vi "TeachableMachines.vi"() -> ()   [LabVIEW 2020]
uses:
  EN1Course-master/_Subs/SystemLink/SL_Subs/SL_XControl.xctl
  EN1Course-master/_Subs/SystemLink/SL_Subs/SystemLink_Write_String.vi
panel:
  in  "Image Path":path
  in  "Path to keras folder":path
  in  "Ask":bool
  in  "stop":bool
  out "dt":u32=141
  out "picture":picture
  out "Percentages":u8[](array[slide])=[0, 99, 1, 0] scale=0.0..100.0
  out "Labels":string="0 go\n1 stop\n2 right\n3 nothing\n"
  in  "SystemLink":T1(xcontrol)
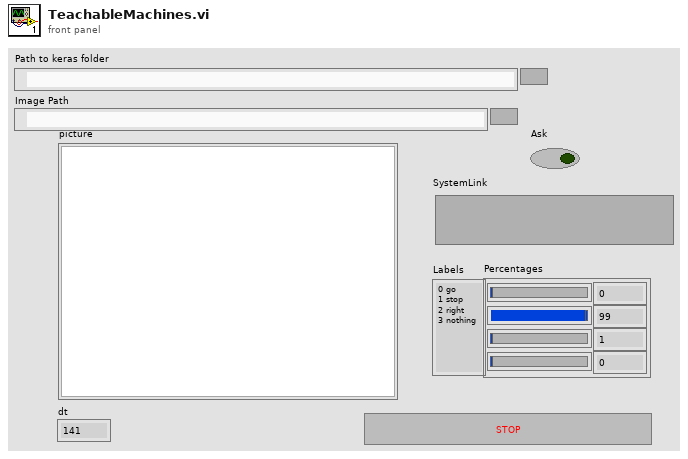
[diagram p1: front panel]
types:
  T1 = cluster{"Tag":string, "Type":string, "Data":string}
  T2 = cluster{"session":refnum<k35>, "Tensor Flow":path, "Image":path, "Labels":string}
  T3 = typedef "imagedata.ctl" = cluster{"image type":i32, "image depth":i32, "image":u8[], "mask":u8[], "colors":u32[], "Rectangle":cluster{"left":i16, "top":i16, "right":i16, "bottom":i16}}
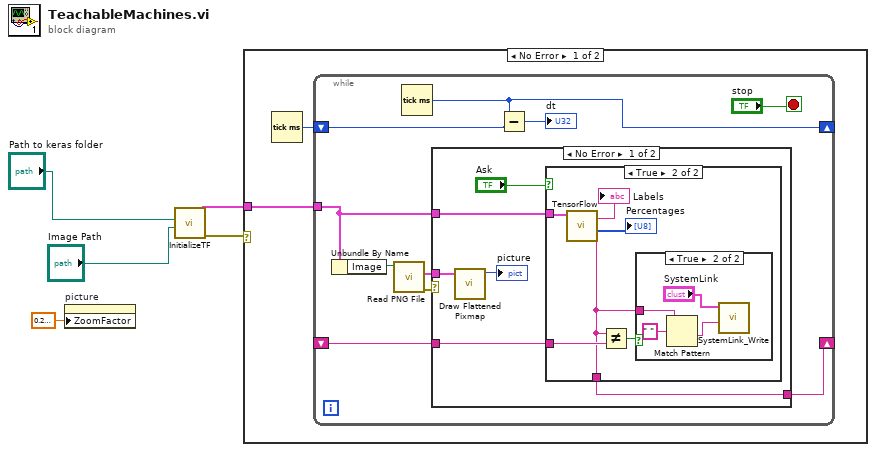
[diagram p0: block diagram]
diagram:
  n1 = property on="picture" class="Pict"("ZoomFactor"=sgl 0.2 ("Zoom Factor")) -> ()  [unwired: 2 in, 2 out]
  n2 = call "InitializeTF.vi"("Image Path"="Image Path", "Path to keras folder"="Path to keras folder") -> ("error out"=w4:errorcluster, "TFinfo out"=w5:T2)  [unwired: 8 in]
  n3 = case shown="No Error" w4 {
    tunnel: w5 -> [w7 _]
    frame No Error {
      n4 = Tick Count (ms)() -> (millisecond timer value=w6:u32)
      n5 = while {
        tunnel: w7 -> [w11]
        shift-right: [w17] -> _
        shift-left: w6 -> [w16]
        shift-right: [w12] -> _
        shift-left: _ -> [w13]
        stop <- "stop" stop-if-true
        n6 = Unbundle By Name(w11) -> ("Image"=w10:path)
        n7 = call <vilib>:"Read PNG File.vi"("path to PNG file"=w10) -> ("error out"=w8:errorcluster, "image data"=w9:T3)  [unwired: 8 in, 1 out]
        n8 = Tick Count (ms)() -> (millisecond timer value=w17:u32)
        n9 = case shown="No Error" w8 {
          tunnel: w13 -> [w23 w35]
          tunnel: [w22 w35] -> w12
          tunnel: w11 -> [w21 _]
          tunnel: w9 -> [w19 _]
          frame No Error {
            n10 = call <vilib>:"Draw Flattened Pixmap.vi"("image data"=w19) -> ("new picture"=→"picture":picture)  [unwired: 8 in]
            n11 = case shown="True" "Ask" {
              tunnel: w23 -> [w24 w29]
              tunnel: [w24 w27] -> w22
              tunnel: w21 -> [_ w25]
              frame False {
              }
              frame True {
                n12 = call "TensorFlow.vi"("TFinfo In"=w25) -> ("Label"=w27:string, "Percentages"=→"Percentages":u8[], "Labels"=→"Labels":string)  [unwired: 6 in, 2 out]
                n13 = Not Equal?(x=w27, y=w29) -> (x != y?=w30:bool)
                n14 = case shown="True" w30 {
                  tunnel: w27 -> [_ w33]
                  frame False {
                  }
                  frame True {
                    n15 = Match Pattern(string=w33, regular expression=" ") -> (after substring=w32:string)  [unwired: 1 in, 3 out]
                    n16 = call-poly "SystemLink_Write.vi"("String"=w32, "SL_XControl"="SystemLink") -> ()  [unwired: 10 in]
                  }
                }
              }
            }
          }
          frame Error {
          }
        }
        n17 = Subtract(x=w17, y=w16) -> (x-y=→"dt":u32)
      }
    }
    frame Error {
    }
  }
